vi "Set Ext Trigger On-Off.vi"(7 "Ext. Trigger":refnum<vi>, 8 "error in":errorcluster, 9 "Head Channel":i16, 10 "Pulsar Handle":i16, 11 "OphirFastX (in)":refnum<k7>) -> (0 "error out":errorcluster, 3 "OphirFastX (out)":refnum<k7>)   [LabVIEW 2009]
panel:
  # "Guillaume Plateau - yguig2@yahoo.fr"
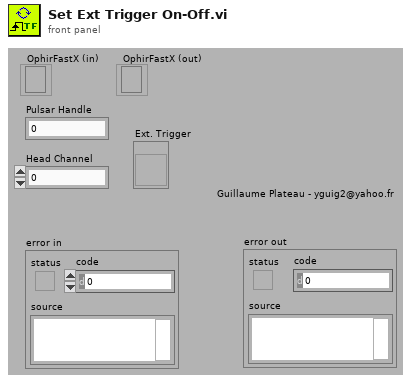
[diagram p1: front panel]
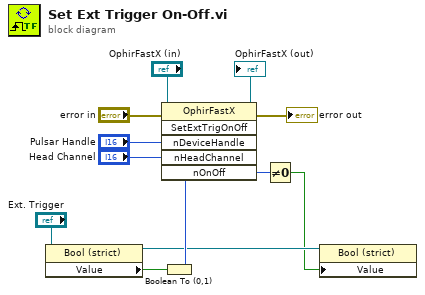
[diagram p0: block diagram]
diagram:
  n1 = property class="Bool (strict)"(reference="Ext. Trigger") -> (reference out=w2:refnum<vi>, "Value"=w3:bool)  [unwired: 1 in, 1 out]
  n2 = Boolean To (0,1)(Boolean=w3) -> (0, 1=w7:i16)
  n3 = invoke class="OphirFastX" method="SetExtTrigOnOff"(reference="OphirFastX (in)", error in="error in", "nDeviceHandle"="Pulsar Handle", "nHeadChannel"="Head Channel", "nOnOff"=w7) -> (reference out=→"OphirFastX (out)":refnum<k7>, error out=→"error out":errorcluster, "nOnOff"=w5:i16)  [unwired: 1 in, 3 out]
  n4 = Not Equal To 0?(x=w5) -> (x != 0?=w1:bool)
  n5 = property class="Bool (strict)"(reference=w2, "Value"=w1) -> ()  [unwired: 1 in, 2 out]
